vi "BPCS Global Variables.vi"() -> ()   [LabVIEW 2018]
panel:
  out "HMI-10TIC100_MA":bool
  out "HMI-10LIC200_MA":bool
  in  "HMI-10TIC100-KPID":dbl[](array[numeric])
  in  "HMI-10HIC100":dbl
  in  "HMI-10TIC100-SP":dbl
  in  "HMI-10HIC200":dbl
  in  "HMI-10LIC200-SP":dbl
  in  "HMI-10LIC200-KPID":dbl[](array[numeric])
  in  "HMI-10HIC300":dbl
  out "BPCS-SIM-TX-ARRAY":dbl[](array[numeric])
  in  "BPCS-10AY300":dbl
  in  "BPCS-10TY100":dbl
  in  "BPCS-10LY200":dbl
  in  "BPCS-10TI100":dbl
  in  "BPCS-10LI200":dbl
  out "SIM-BPCS-RX-ARRAY":dbl[](array[numeric])
  out "SIS-BPCS-RX-Array":bool[](array[boolean])
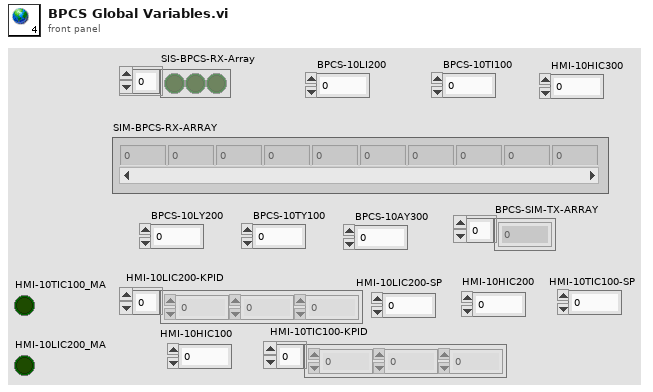
[diagram p1: front panel]
diagram:
